vi "TCP-Send Command (byte array) Receive I32.vi"(0 "PXI Address":string, 5 "Port":i32, 7 "Command":string, 9 "timeout (ms)":i32=5000, 11 "error in (no error)":errorcluster) -> (4 "value":i32, 10 "result":i32, 15 "error out":errorcluster)   [LabVIEW 2020]
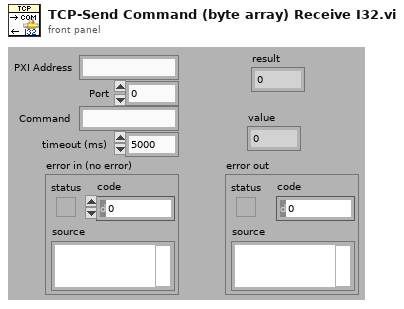
[diagram p1: front panel]
types:
  T1 = enum16{"Standard", "Buffered", "CRLF", "Immediate"}
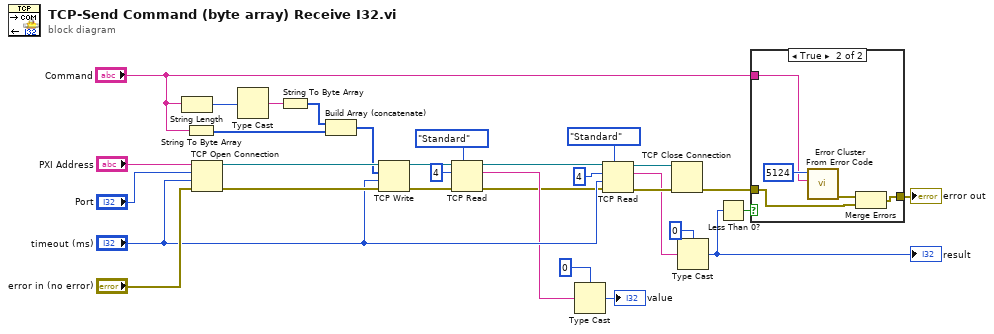
[diagram p0: block diagram]
diagram:
  n1 = String Length(string="Command") -> (length=w8:i32)
  n2 = String To Byte Array(string="Command") -> (unsigned byte array=w9:u8[])
  n3 = TCP Open Connection(address="PXI Address", remote port or service name="Port", timeout ms (60000)="timeout (ms)", error in (no error)="error in (no error)") -> (connection ID=w27:refnum<k5>, error out=w28:errorcluster)  [unwired: 1 in]
  n4 = Type Cast(x=w8) -> (*(type *) &x=w7:string)  [unwired: 1 in]
  n5 = String To Byte Array(string=w7) -> (unsigned byte array=w6:u8[])
  n6 = Build Array (concatenate)(w6, w9) -> (w4:u8[])
  n7 = TCP Write(connection ID=w27, data in=w4, error in (no error)=w28, 9:"timeout (ms)") -> (connection ID out=w16:refnum<k5>, error out=w15:errorcluster)  [unwired: 1 out]
  n8 = TCP Read(connection ID=w16, bytes to read=4, error in (no error)=w15, 7:T1."Standard" ("mode (standard)")) -> (connection ID out=w14:refnum<k5>, data out=w13:string, error out=w12:errorcluster)  [unwired: 1 in]
  n9 = Type Cast(type=0, x=w13) -> (*(type *) &x=→"value":i32)
  n10 = TCP Read(connection ID=w14, bytes to read=4, error in (no error)=w12, 7:T1."Standard" ("mode (standard)"), 9:"timeout (ms)") -> (connection ID out=w23:refnum<k5>, data out=w22:string, error out=w24:errorcluster)
  n11 = TCP Close Connection(connection ID=w23, error in (no error)=w24) -> (error out=w17:errorcluster)  [unwired: 1 in, 1 out]
  n12 = Type Cast(type=0, x=w22) -> (*(type *) &x=w20:i32)
  "result" <- w20
  n13 = Less Than 0?(x=w20) -> (x < 0?=w19:bool)
  n14 = case shown="True" w19 {
    tunnel: [w32 w34] -> w18
    tunnel: w17 -> [w32 w33]
    tunnel: "Command" -> [_ w35]
    frame False {
    }
    frame True {
      n15 = call <vilib>:"Error Cluster From Error Code.vi"("error message (\"\")"=w35, "error code (0)"=5124) -> ("error out"=w37:errorcluster)  [unwired: 7 in]
      n16 = Merge Errors(w37, w33) -> (w34:errorcluster)
    }
  }
  "error out" <- w18
